vi "ILABW_ViStatus.vi"(2 "errorIn":errorcluster, 3 "name":string) -> (0 "errorOut":string, 1 "status":i32)   [LabVIEW 2012]
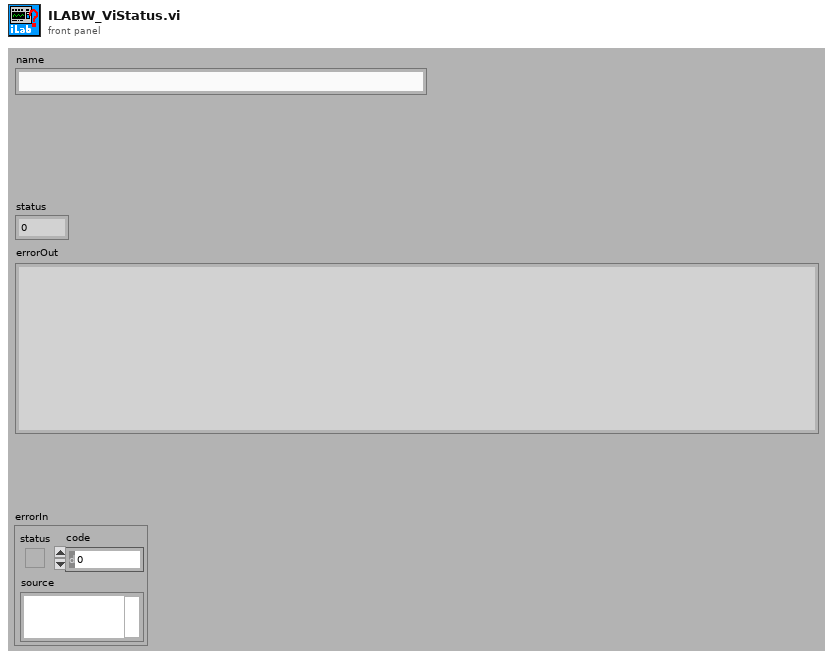
[diagram p1: front panel]
types:
  T1 = enum32{"Bad", "Idle", "Run top level", "Running"}
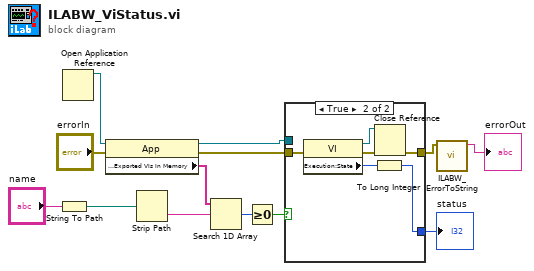
[diagram p0: block diagram]
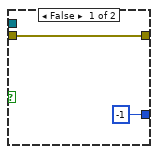
[diagram p2: hidden frame]
diagram:
  n1 = String To Path(string="name") -> (path=w5:path)
  n2 = Open Application Reference() -> (3:w7:refnum<vi>)  [unwired: 4 in, 1 out]
  n3 = property class="App"(reference=w7, error in="errorIn") -> (reference out=w10:refnum<vi>, error out=w3:errorcluster, "Application:Exported VIs In Memory"=w13:string[])
  n4 = Strip Path(path=w5) -> (name=w4:string)  [unwired: 1 out]
  n5 = Search 1D Array(1D array=w13, element=w4) -> (index of element=w12:i32)  [unwired: 1 out]
  n6 = Greater Or Equal To 0?(x=w12) -> (x >= 0?=w11:bool)
  n7 = case shown="True" w11 {
    tunnel: w3 -> [w15 w16]
    tunnel: w10 -> [_ _]
    tunnel: [w15 w17] -> w2
    tunnel: [-1 w20] -> w9
    frame False {
    }
    frame True {
      n8 = property class="VI"(error in=w16) -> (reference out=w19:refnum<vi>, error out=w18:errorcluster, "Execution:State"=w21:T1)  [unwired: 1 in]
      n9 = To Long Integer(number=w21) -> (32bit integer=w20:i32)
      n10 = Close Reference(reference=w19, error in (no error)=w18) -> (error out=w17:errorcluster)
    }
  }
  "status" <- w9
  n11 = call "ILABW_ErrorToString.vi"("errorIn"=w2) -> ("errorOut"=→"errorOut":string)  [unwired: 10 in]
